vi "Read Setup File.vi"(8 "error in (no error)":errorcluster, 11 "JSON in":refnum<class "JSON.lvclass">) -> (0 "error out":errorcluster, 3 "JSON out":refnum<class "JSON.lvclass">)   [LabVIEW 2018, in "JSON.lvclass"]
uses:
  JSON.lvclass
  JSON.lvclass/JSON.ctl
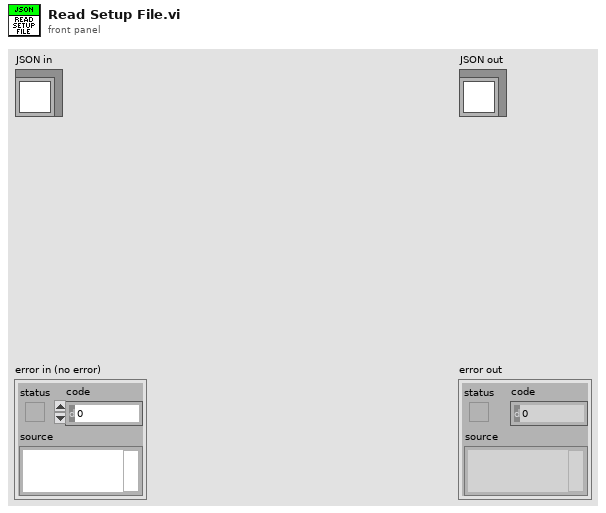
[diagram p1: front panel]
types:
  T1 = enum16{"open", "replace", "create", "open or create", "replace or create", "replace or create with confirmation"}
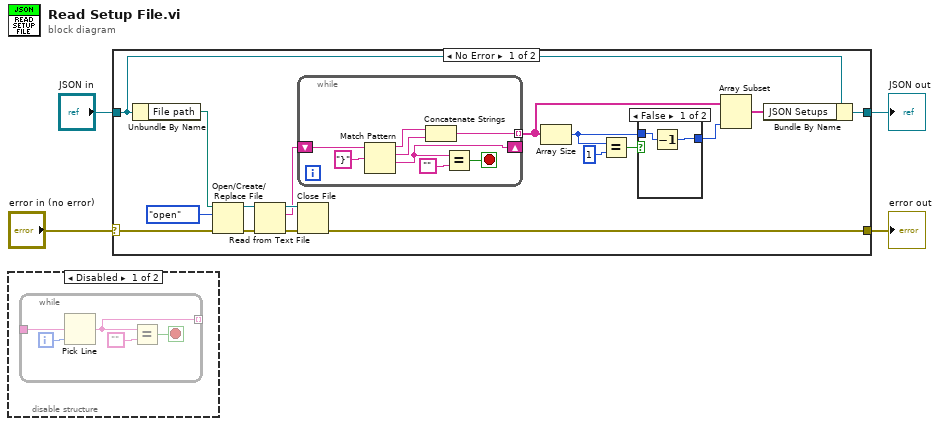
[diagram p0: block diagram]
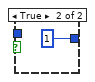
[diagram p3: hidden frame]
diagram:
  n1 = disable-structure shown="Disabled" {
    frame Disabled {
      n2 = while {
        tunnel: [w6] -> _ mode=indexing
        tunnel: _ -> [w5]
        i -> [w9]
        stop <- w7 stop-if-true
        n3 = Pick Line(multi-line string=w5, line index=w9) -> (output string=w6:string)  [unwired: 1 in]
        n4 = Equal?(x=w6, y="") -> (x = y?=w7:bool)
      }
    }
    frame Enabled {
    }
  }
  n5 = case shown="No Error" "error in (no error)" {
    selector: "error in (no error)" -> [w25 w39]
    tunnel: [w20 w39] -> w3
    tunnel: [w18 w38] -> w1
    tunnel: "JSON in" -> [w19 w38]
    frame No Error {
      n6 = Unbundle By Name(w19) -> ("File path"=w17:path)
      n7 = Open/Create/Replace File(file path (use dialog)=w17, error in=w25, operation (0:open)=T1."open") -> (refnum out=w22:refnum<file>, error out=w24:errorcluster)  [unwired: 3 in, 1 out]
      n8 = Read from Text File(file (use dialog)=w22, error in=w24) -> (refnum out=w21:refnum<file>, text=w16:string, error out=w23:errorcluster)  [unwired: 2 in, 1 out]
      n9 = while {
        shift-right: [w30] -> _
        shift-left: w16 -> [w34]
        tunnel: [w31] -> w15 mode=indexing
        stop <- w36 stop-if-true
        n10 = Match Pattern(string=w34, regular expression="}" ("search string/char (-)")) -> (before substring=w33:string, match substring=w32:string, after substring=w30:string)  [unwired: 1 in, 1 out]
        n11 = Concatenate Strings(w33, w32) -> (w31:string)
        n12 = Equal?(x=w30, y="") -> (x = y?=w36:bool)
      }
      n13 = Close File(refnum=w21, error in=w23) -> (error out=w20:errorcluster)  [unwired: 1 out]
      n14 = Array Size(array=w15) -> (size(s)=w10:i32)
      n15 = Equal?(x=w10, y=1) -> (x = y?=w13:bool)
      n16 = case shown="False" w13 {
        tunnel: [w27 1] -> w11
        tunnel: w10 -> [w28 _]
        frame False {
          n17 = Decrement(x=w28) -> (x-1=w27:i32)
        }
        frame True {
        }
      }
      n18 = Array Subset(array=w15, length=w11) -> (w14:string[])  [unwired: 1 in]
      n19 = Bundle By Name(cluster=w19, "JSON Setups"=w14) -> (w18:refnum<class "JSON.lvclass">)
    }
    frame Error {
    }
  }
  "error out" <- w3
  "JSON out" <- w1
